vi "Task Uninit.vi"(8 "error in (no error)":errorcluster, 11 "DebugGUI in":refnum<class "DebugGUI.lvclass">) -> (0 "error out":errorcluster, 3 "DebugGUI out":refnum<class "DebugGUI.lvclass">)   [LabVIEW 2020, in "Volatus.lvlib" / "DebugGUI.lvclass"]
uses:
  DebugGUI.lvclass
  DebugGUI.lvclass/DebugGUI.ctl
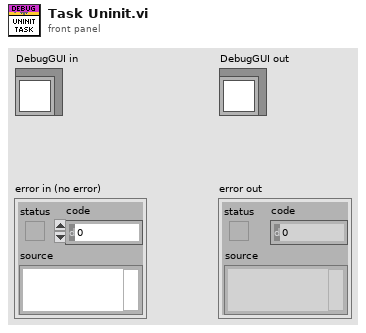
[diagram p1: front panel]
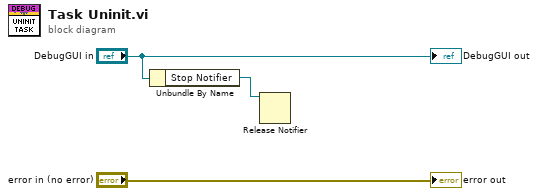
[diagram p0: block diagram]
diagram:
  n1 = Unbundle By Name("DebugGUI in") -> ("Stop Notifier"=w1:refnum<notifier>)
  n2 = Release Notifier(notifier=w1) -> ()  [unwired: 2 in, 3 out]
  "error out" <- "error in (no error)"
  "DebugGUI out" <- "DebugGUI in"
